vi "Position_show_and_move.vi"(6 "Target position":dbl[](array[numeric]), 7 "Measurement running":bool, 8 "error in":errorcluster, 9 "System no.":i32, 10 "Move":bool, 11 "actual scan position":dbl[](array[numeric])) -> (0 "error out":errorcluster, 3 "Value":dbl[](array[numeric]))   [LabVIEW 2009]
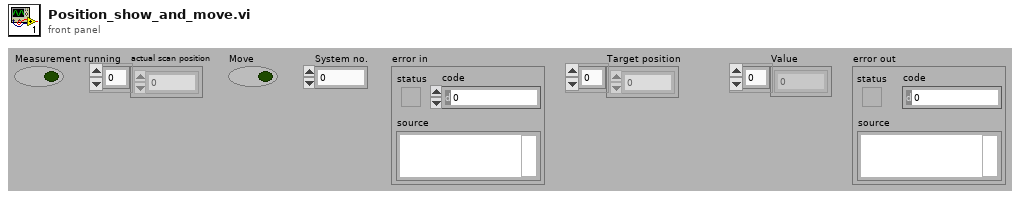
[diagram p1: front panel]
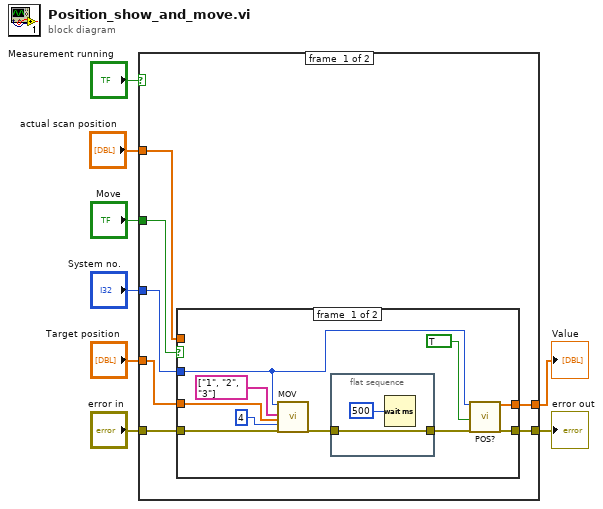
[diagram p0: block diagram]
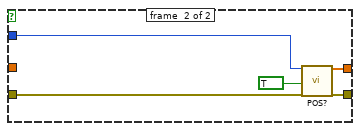
[diagram p2: hidden frame]
diagram:
  n1 = case shown="False" "Measurement running" {
    tunnel: [w15 w34] -> w8
    tunnel: "error in" -> [w14 w34]
    tunnel: "System no." -> [w13 _]
    tunnel: "Move" -> [w12 _]
    tunnel: "Target position" -> [w11 _]
    tunnel: "actual scan position" -> [w10 w33]
    tunnel: [w9 w33] -> w7
    frame #0 {
      n2 = case shown="False" w12 {
        tunnel: [w20 w32] -> w15
        tunnel: w14 -> [w25 w30]
        tunnel: w13 -> [w19 w29]
        tunnel: [w18 w28] -> w9
        tunnel: w11 -> [w23 _]
        tunnel: w10 -> [_ _]
        frame #0 {
          n3 = call <userlib>:"MOV.vi"("System no."=w19, "Axes to move"=string[] ["1", "2", "3"], "Position values"=w23, "No.of digits"=i16 4, "error in"=w25) -> ("error out"=w17:errorcluster)  [unwired: 14 out]
          n4 = flat-sequence {
            tunnel: w17 -> [w27]
            tunnel: [w27] -> w16
            frame #0 {
              n5 = Wait (ms)(milliseconds to wait=u32 500) -> ()  [unwired: 1 out]
            }
          }
          n6 = call <userlib>:"POS?.vi"("System no."=w19, "All axes?"=TRUE, "error in"=w16) -> ("Position"=w18:dbl[], "error out"=w20:errorcluster)  [unwired: 2 in, 13 out]
        }
        frame #1 {
          n7 = call <userlib>:"POS?.vi"("System no."=w29, "All axes?"=TRUE, "error in"=w30) -> ("Position"=w28:dbl[], "error out"=w32:errorcluster)  [unwired: 2 in, 13 out]
        }
      }
    }
    frame #1 {
    }
  }
  "error out" <- w8
  "Value" <- w7
